vi "Add Nested Tag.vi"(5 "Name (Optional)":string, 7 "ID":u32, 8 "error in (no error)":errorcluster, 9 "Tag":refnum<class "Basic Type.lvclass">, 10 "Parent Message Path (This)":cluster{"Tag ID / Name":variant, "Index":i32}[](array[cluster]), 11 "Raw Message in":refnum<class "Raw Message.lvclass">) -> (0 "error out":errorcluster, 3 "Raw Message out":refnum<class "Raw Message.lvclass">)   [LabVIEW 2020, in "Protobuf RAW.lvlib" / "Raw Message.lvclass"]
uses:
  Raw Message.lvclass
  Raw Message.lvclass/Raw Message.ctl
  E:/Labview/LV 2020/Libs/LV Protobuf Raw/Source/Tag/Basic Type.lvclass
  E:/Labview/LV 2020/Libs/LV Protobuf Raw/Source/Proto Value/Proto Type.lvclass
  E:/Labview/LV 2020/Libs/LV Protobuf Raw/Source/Type Serializer/Type Serializer.lvclass
  E:/Labview/LV 2020/Libs/LV Protobuf Raw/Source/String Representable/String Representable.lvclass
  E:/Labview/LV 2020/Libs/LV Protobuf Raw/Source/Wire Type Group/Wire Type Group.lvclass
  E:/Labview/LV 2020/Libs/LV Protobuf Raw/Source/LEN Encoder/LEN.lvclass
  E:/Labview/LV 2020/Libs/LV Protobuf Raw/Source/Message/Raw Message.lvclass
  Tag/Basic Type.lvclass
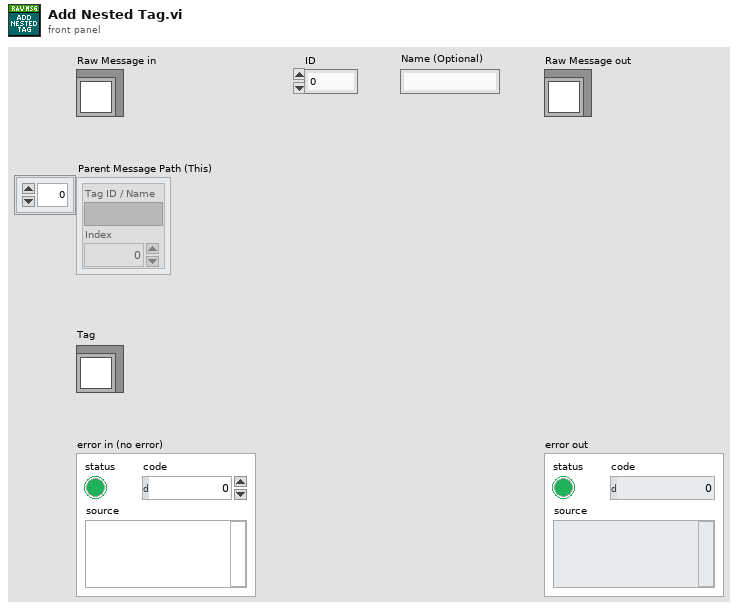
[diagram p1: front panel]
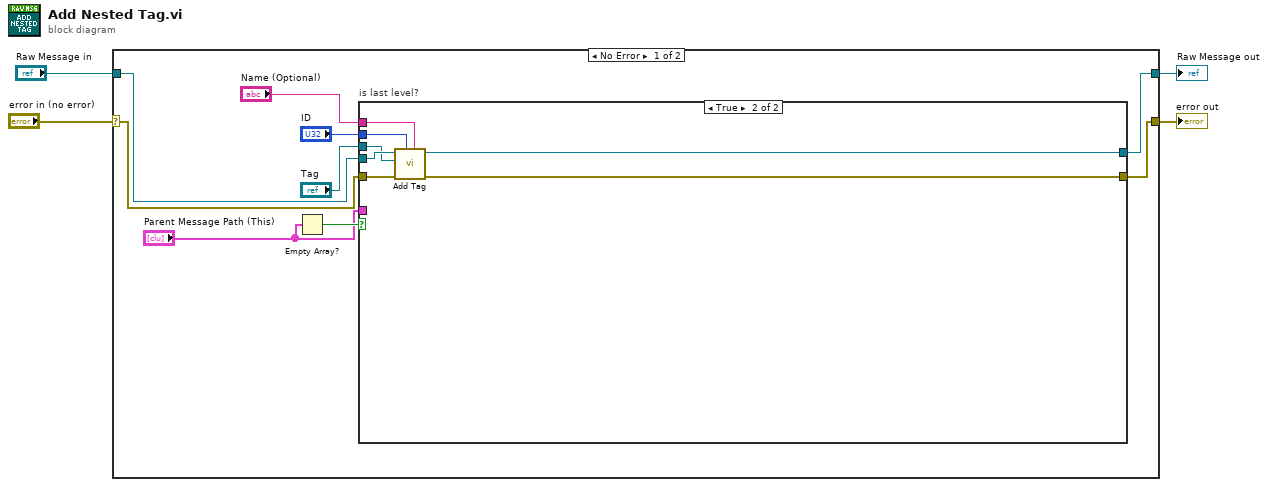
[diagram p0: block diagram]
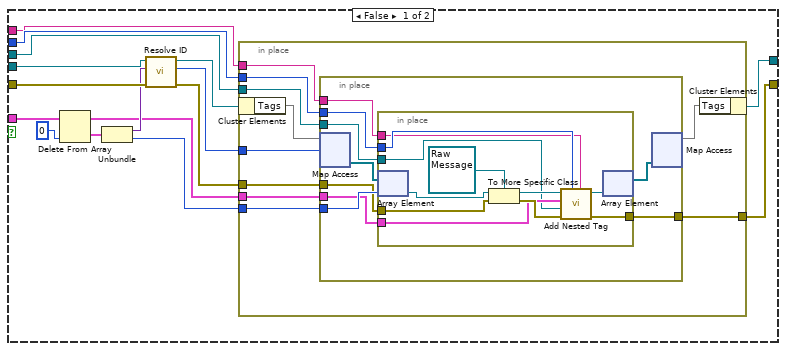
[diagram p2: hidden frame]
diagram:
  n1 = case shown="No Error" "error in (no error)" {
    selector: "error in (no error)" -> [w10 w67]
    tunnel: [w8 w67] -> w4
    tunnel: [w13 _] -> w1
    tunnel: "Raw Message in" -> [w9 _]
    frame No Error {
      n2 = Empty Array?(array="Parent Message Path (This)") -> (empty?=w12:bool)
      n3 = case "is last level?" shown="True" w12 {
        tunnel: [w29 w65] -> w13
        tunnel: [w28 w66] -> w8
        tunnel: "Tag" -> [w27 w60]
        tunnel: w10 -> [w26 w63]
        tunnel: w9 -> [w25 w64]
        tunnel: "Parent Message Path (This)" -> [w19 _]
        tunnel: "ID" -> [w15 w62]
        tunnel: "Name (Optional)" -> [w14 w61]
        frame False {
          n4 = Delete From Array(array=w19, index=0) -> (deleted portion=w18:cluster{"Tag ID / Name":variant, "Index":i32}, array with subset deleted=w17:cluster{"Tag ID / Name":variant, "Index":i32}[])  [unwired: 1 in]
          n5 = Unbundle(w18) -> ("Tag ID / Name"=w21:variant, "Index"=w20:i32)
          n6 = call "Resolve ID.vi"("error in (no error)"=w26, "Tag ID / Name"=w21, "Raw Message in"=w25) -> ("error out"=w24:errorcluster, "Tag ID"=w23:u32, "Raw Message out"=w22:refnum<class "Raw Message.lvclass">)  [unwired: 6 in]
          n7 = in-place {
            in-place-border: w23 -> [w37]
            in-place-border: w20 -> [w36]
            in-place-border: w24 -> [w35]
            in-place-border: w17 -> [w34]
            in-place-border: [w33] -> w28
            in-place-border: w27 -> [w32]
            in-place-border: w15 -> [w31]
            in-place-border: w14 -> [w30]
            n8 = in-place-cluster #1(w22) -> ("Tags"=w39:map{u32, refnum<class "Basic Type.lvclass">[]})
            n9 = in-place {
              in-place-border: w36 -> [w46]
              in-place-border: w35 -> [w45]
              in-place-border: w34 -> [w44]
              in-place-border: [w43] -> w33
              in-place-border: w32 -> [w42]
              in-place-border: w31 -> [w41]
              in-place-border: w30 -> [w40]
              n10 = in-place-map #2(w39, w37) -> (w48:refnum<class "Basic Type.lvclass">[])  [unwired: 1 in, 1 out]
              n11 = in-place {
                in-place-border: w45 -> [w55]
                in-place-border: w44 -> [w54]
                in-place-border: [w52] -> w43
                in-place-border: w42 -> [w51]
                in-place-border: w41 -> [w50]
                in-place-border: w40 -> [w49]
                n12 = in-place-array #3(w48, w46) -> (w59:refnum<class "Basic Type.lvclass">)
                n13 = To More Specific Class(target class=refnum<class "Raw Message.lvclass"> refnum ("Raw Message out"), reference=w59, error in=w55) -> (specific class reference=w58:refnum<class "Raw Message.lvclass">, error out=w57:errorcluster)
                n14 = call "Add Nested Tag.vi"("Name (Optional)"=w49, "ID"=w50, "error in (no error)"=w57, "Tag"=w51, "Parent Message Path (This)"=w54, "Raw Message in"=w58) -> ("error out"=w52:errorcluster, "Raw Message out"=w53:refnum<class "Raw Message.lvclass">)  [unwired: 4 in]
                n15 = in-place-array #3(w53) -> (w47:refnum<class "Basic Type.lvclass">[])  [unwired: 1 out]
              }
              n16 = in-place-map #2(w47) -> (w38:map{u32, refnum<class "Basic Type.lvclass">[]})  [unwired: 1 in, 2 out]
            }
            n17 = in-place-cluster #1("Tags"=w38) -> (w29:refnum<class "Raw Message.lvclass">)
          }
        }
        frame True {
          n18 = call-dynamic "Add Tag.vi"("Name (Optional)"=w61, "ID"=w62, "error in (no error)"=w63, "Tag Value"=w60, "Message in"=w64) -> ("error out"=w66:errorcluster, "Message out"=w65:refnum<class "Raw Message.lvclass">)  [unwired: 5 in]
        }
      }
    }
    frame Error {
    }
  }
  "error out" <- w4
  "Raw Message out" <- w1
